vi "HW Config.vi"() -> ()   [LabVIEW 2018]
uses:
  Subvi/Global.vi
panel:
  in  "Bar":bool
  in  "退出 3":bool
  in  "另存为":bool
  in  "保存":bool
  in  "open":bool
  in  "新建":bool
  in  "delete":bool
  in  "add":bool
  out "布尔":bool
  in  "Add":bool
  in  "Tree":string(tree)="DSO-2250 USB"
  out "Ready":u8(slide) max=101 scale=0.0..100.0
  in  "File Name":string caption="文件名称"
  in  "Save As":bool
  in  "Save":bool
  in  "Multicolumn Listbox":i32(listbox)=-1
  # "添加：选中右边你要插入的行，然后双击获点击“添加(F1)”左边你的设备\n即可添加到右边所选中行的前面\n删除：选中右边你要删除的行，点击\"删除（DEL）\"\n！"
  # "DEMO:V0.0.1"
  # "ID"
  # "准备就绪"
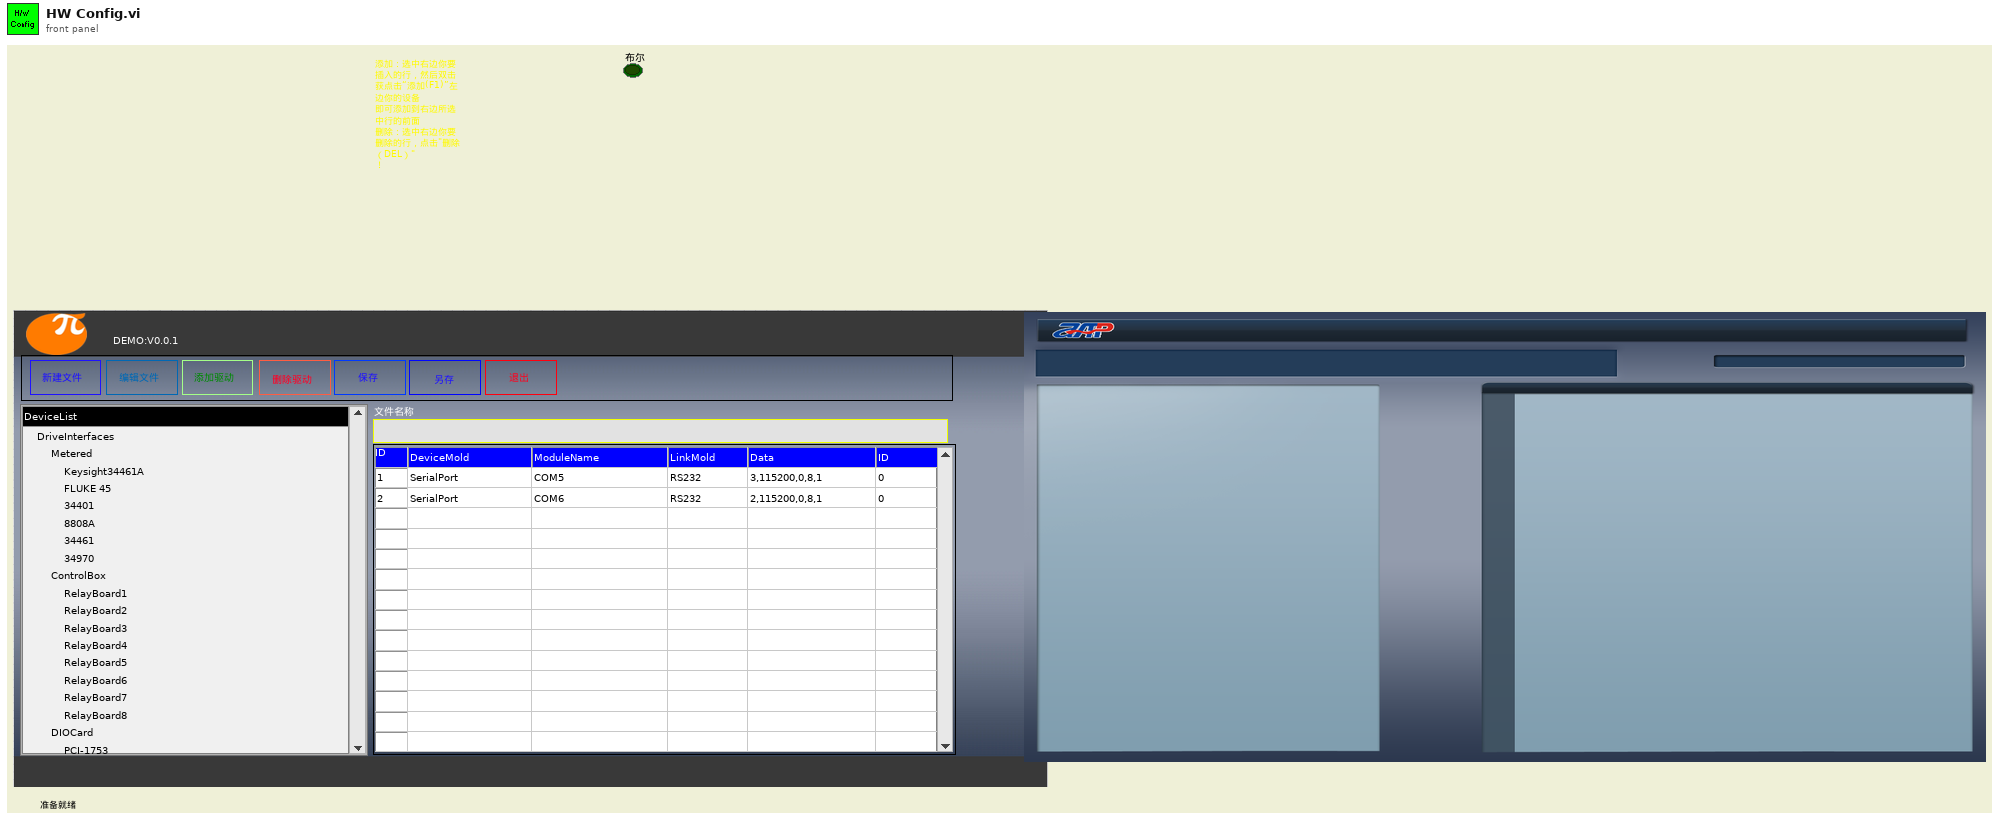
[diagram p1: front panel]
types:
  T1 = enum16{"open", "replace", "create", "open or create", "replace or create", "replace or create with confirmation"}
  T2 = typedef "Window Refnum.ctl" = refnum<k1>
  T3 = typedef "Window Rectangle.ctl" = cluster{"left":i16, "top":i16, "right":i16, "bottom":i16}
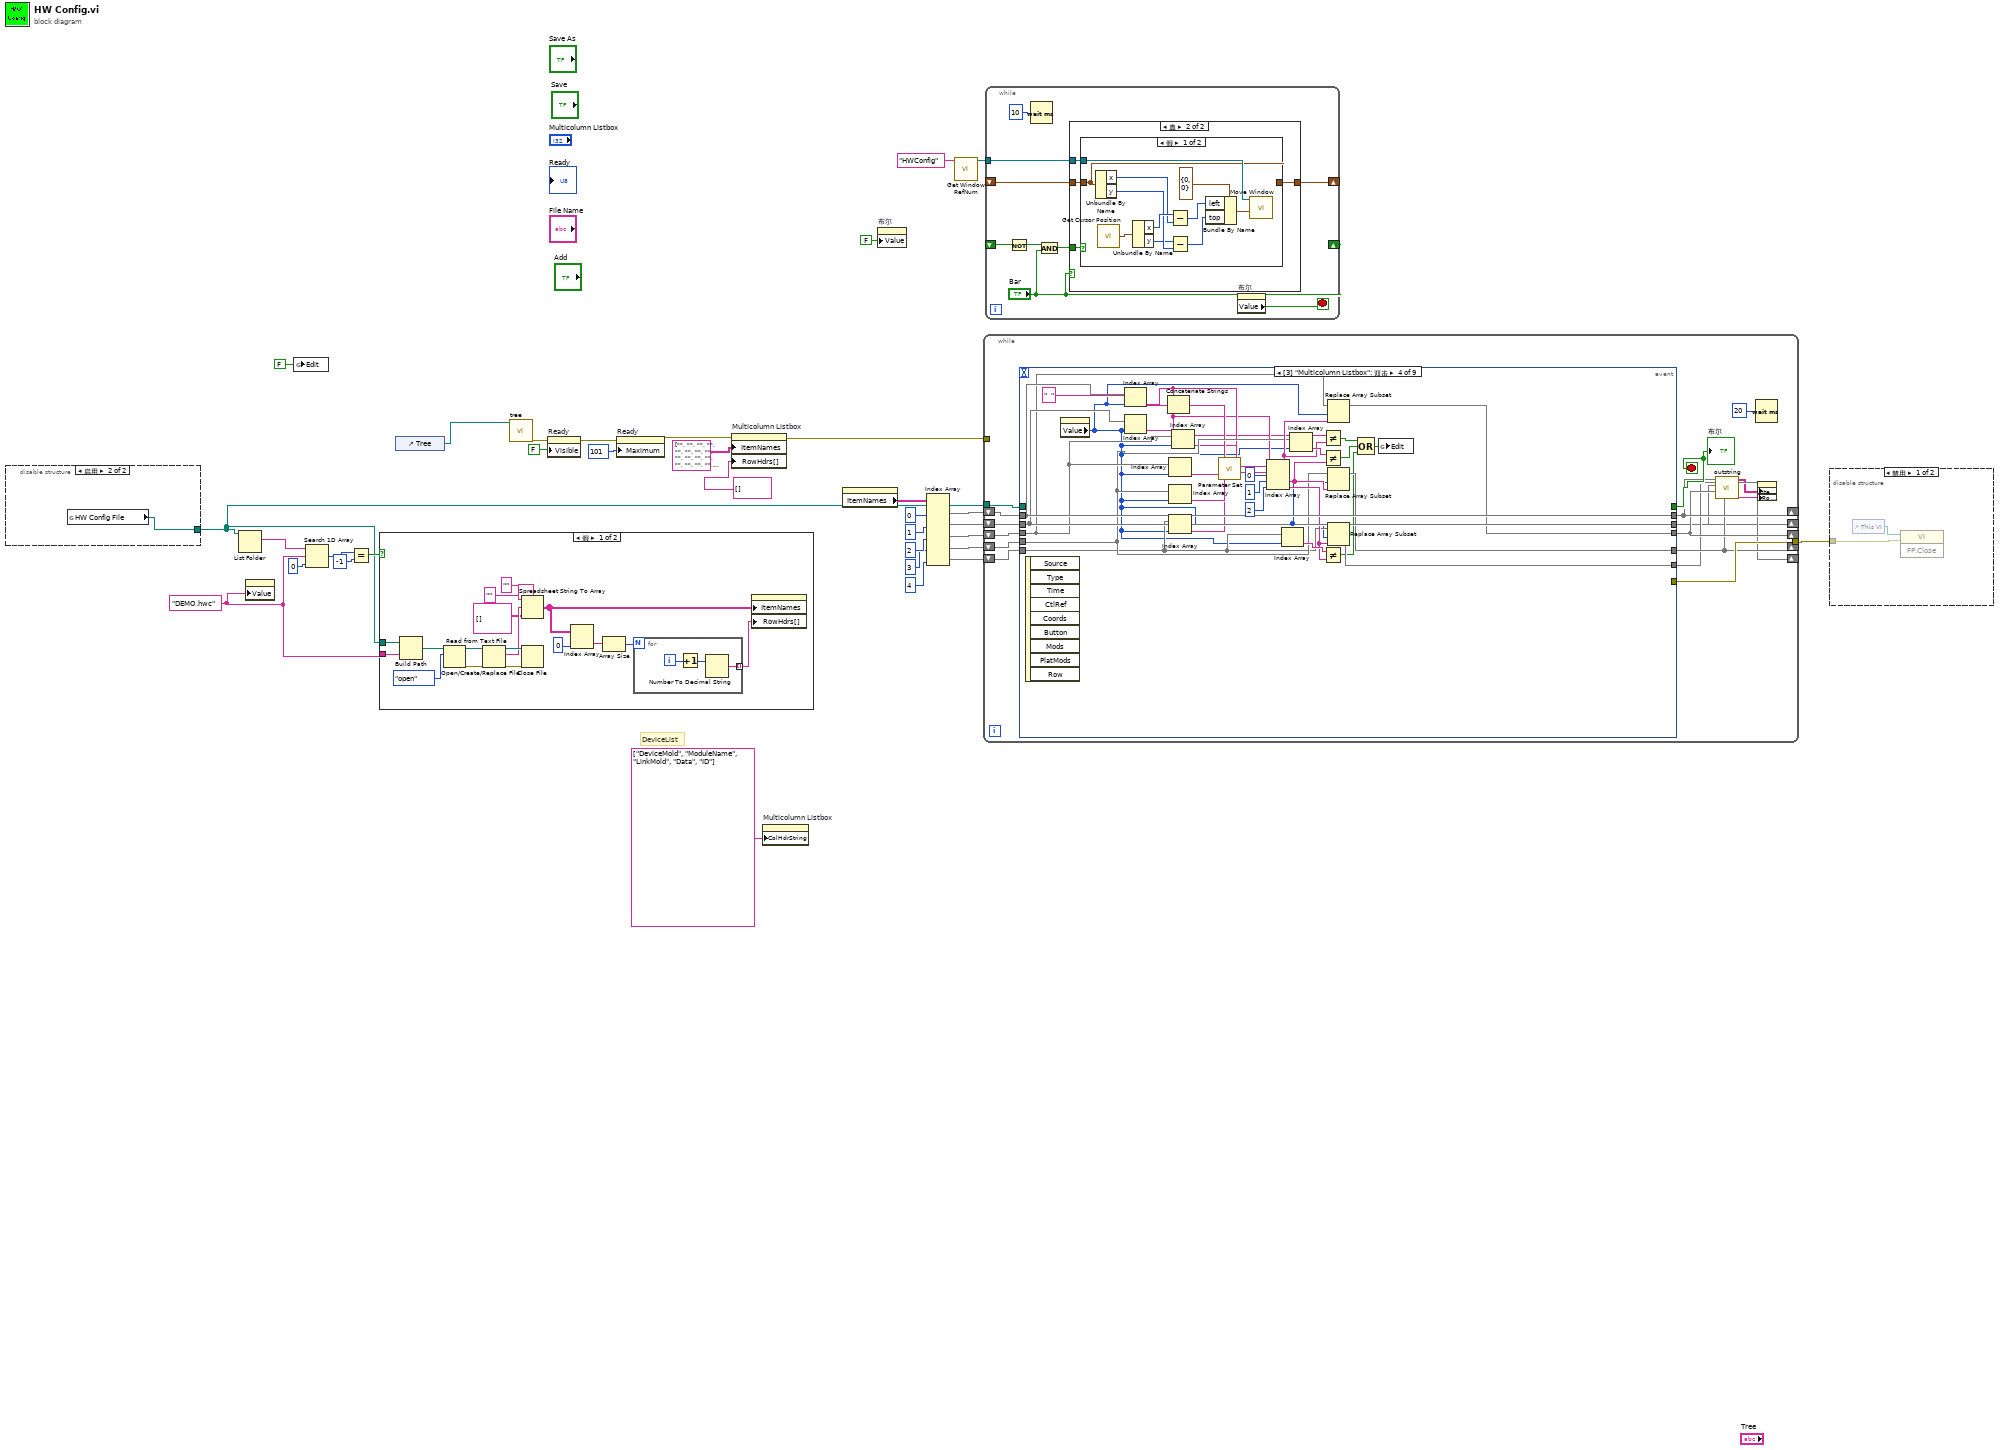
[diagram p0: block diagram]
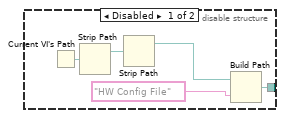
[diagram p3: hidden frame]
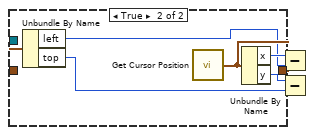
[diagram p5: hidden frame]
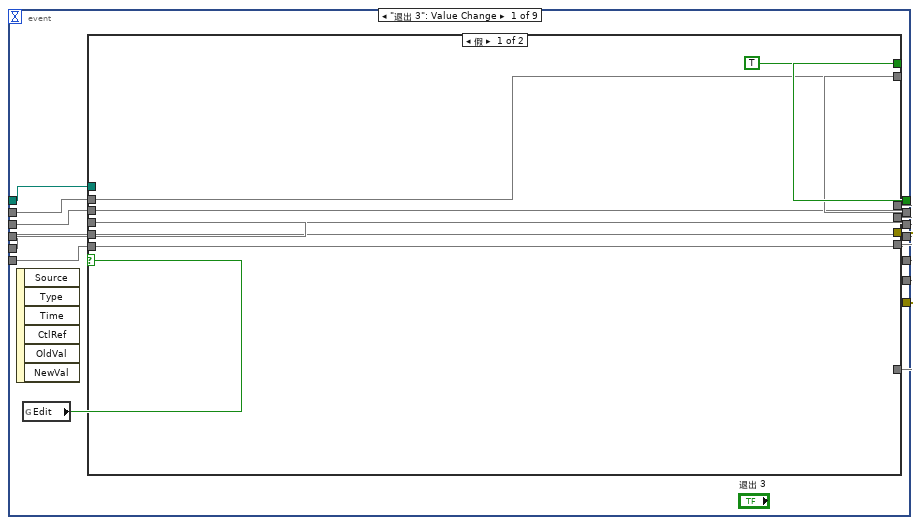
[diagram p6: hidden frame]
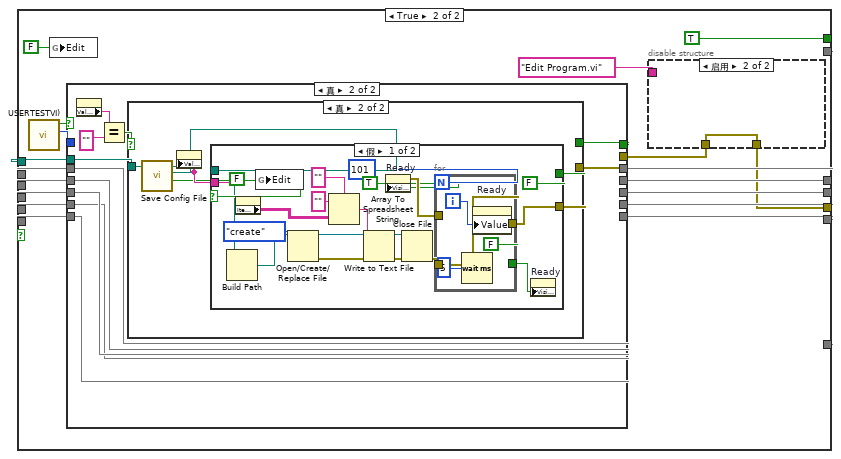
[diagram p7: hidden frame]
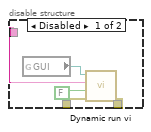
[diagram p8: hidden frame]
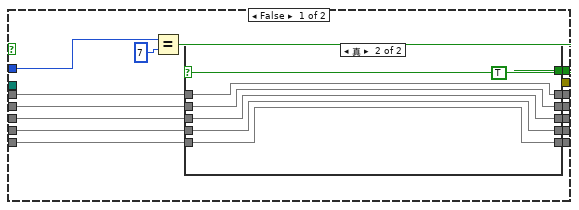
[diagram p9: hidden frame]
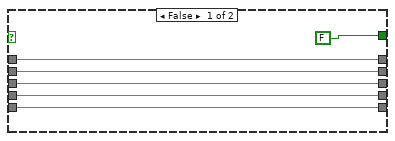
[diagram p10: hidden frame]
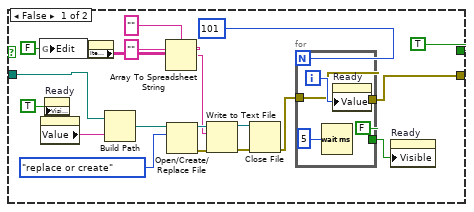
[diagram p11: hidden frame]
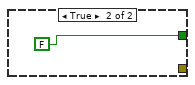
[diagram p12: hidden frame]
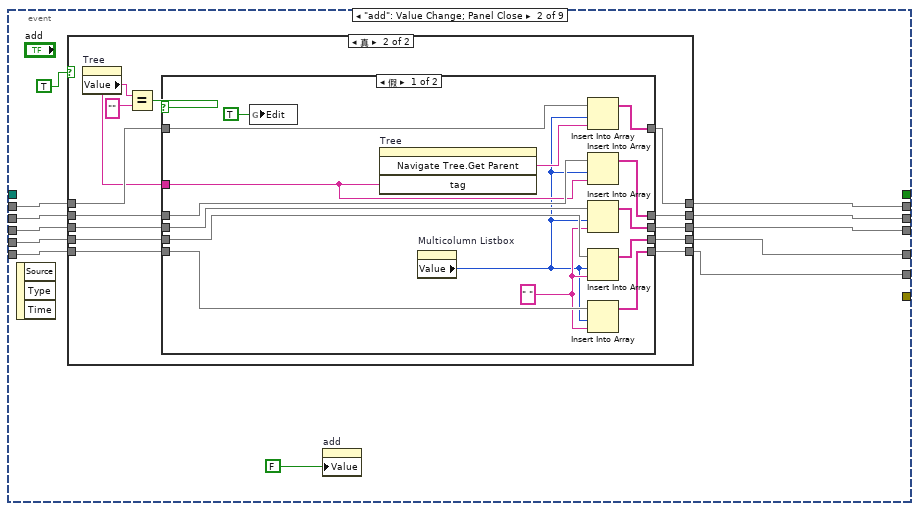
[diagram p13: hidden frame]
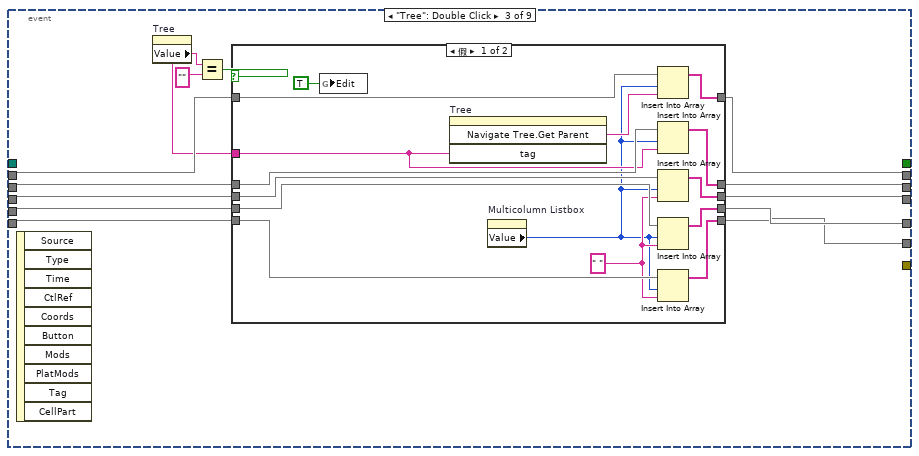
[diagram p16: hidden frame]
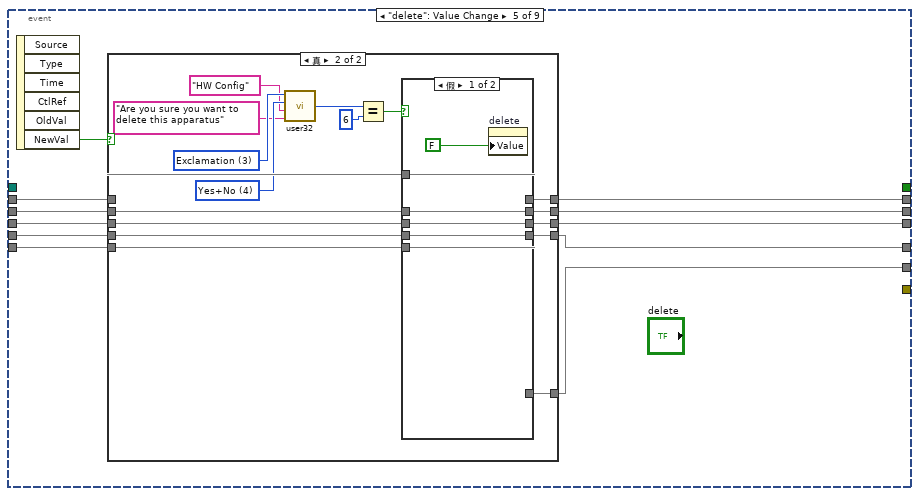
[diagram p18: hidden frame]
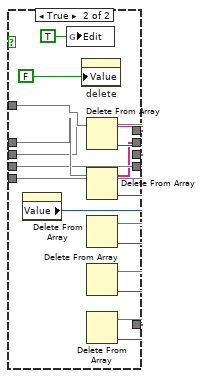
[diagram p20: hidden frame]
diagram:
  w25 = "DEMO.hwc" ("element")
  # "DeviceList"
  n1 = disable-structure shown="启用" {
    disable-tunnel: [w35 w39] -> w19
    frame Disabled {
      n2 = Current VI's Path() -> (path=w34:path)
      n3 = Strip Path(path=w34) -> (stripped path=w37:path)  [unwired: 1 out]
      n4 = Strip Path(path=w37) -> (stripped path=w38:path)  [unwired: 1 out]
      n5 = Build Path(base path=w38, name or relative path="HW Config File") -> (appended path=w35:path)
    }
    frame Enabled {
      n6 = global read "Global.vi" "HW Config File"() -> (w39:path)
    }
  }
  n7 = List Folder(path=w19) -> (filenames=w20:string[])  [unwired: 1 in, 5 out]
  n8 = property on="File Name" class="Str"("Value"=w25) -> ()  [unwired: 2 in, 2 out]
  n9 = global write "Global.vi" "Edit"(FALSE) -> ()
  n10 = Search 1D Array(1D array=w20, element=w25, start index (0)=0) -> (index of element=w22:i32)
  n11 = Equal?(x=w22, y=-1) -> (x = y?=w24:bool)
  n12 = case shown="假" w24 {
    tunnel: w19 -> [w56 w68]
    tunnel: w25 -> [w55 w67]
    frame False {
      n13 = Build Path(base path=w56, name or relative path=w55) -> (appended path=w54:path)
      n14 = Open/Create/Replace File(file path (use dialog)=w54, operation (0:open)=T1."open") -> (refnum out=w53:refnum<file>, error out=w51:errorcluster)  [unwired: 1 in, 4 out]
      n15 = Read from Text File(file (use dialog)=w53, error in=w51) -> (refnum out=w52:refnum<file>, text=w48:string, error out=w50:errorcluster)  [unwired: 3 out]
      n16 = Spreadsheet String To Array(delimiter (Tab)="", format string="", spreadsheet string=w48, array type (2D Dbl)=string[][] []) -> (array=w44:string[][])
      n17 = Close File(refnum=w52, error in=w50) -> ()  [unwired: 2 out]
      n18 = Index Array(array=w44, index (col)=0 ("disabled index (col)")) -> (element=w42:string[])  [unwired: 1 in]
      n19 = Array Size(array=w42) -> (size(s)=w41:i32)
      n20 = for {
        N: w41 -> [_]
        tunnel: [w57] -> w40 mode=indexing
        i -> [w59]
        n21 = Increment(x=w59) -> (x+1=w58:i32)
        n22 = Number To Decimal String(number=w58) -> (decimal integer string=w57:string)  [unwired: 1 out]
      }
      n23 = property on="Multicolumn Listbox" class="MCListbox (严格)"("ItemNames"=w44, "RowHdrs[]"=w40) -> ()  [unwired: 2 in, 2 out]
    }
    frame True {
      n24 = Build Path(base path=w68, name or relative path=w67) -> (appended path=w66:path)
      n25 = Open/Create/Replace File(file path (use dialog)=w66, operation (0:open)=T1."create") -> (refnum out=w64:refnum<file>, error out=w63:errorcluster)  [unwired: 1 in, 4 out]
      n26 = Write to Text File(file (use dialog)=w64, text="DC Source\tAPM\tRS 232\t2,9600,0,8,1\t1\nDC Source\tAPM\tRS 232\t3,9600,0,8,1\t2\nDC Source\tAPM\tRS 232\t4,9600,0,8,1\t3\nDC Source\tAPM\tRS 232\t5,9600,0,8,1\t4\nOscilloscope\tDSO-2250 USB\tUSB\t0\t1\nCAN Card\tGY8507\tUSB\t0\t1\nDIO Card\tPCI 1753\tPCI Card\t4\t1\nDAQ\tPCI-1713\tPCI Card\t3\t1\n", error in=w63) -> (refnum out=w62:refnum<file>, error out=w61:errorcluster)  [unwired: 2 out]
      n27 = Close File(refnum=w62, error in=w61) -> ()  [unwired: 2 out]
    }
  }
  n28 = control-ref of="Tree"() -> (w4:refnum<vi>)
  n29 = call "tree.vi"("search"=w4) -> ("error out"=w3:errorcluster)  [unwired: 9 in, 1 out]
  n30 = property on="Ready" class="Slide (严格)"(error in=w3, "Visible"=FALSE) -> (error out=w27:errorcluster)  [unwired: 1 in, 1 out]
  n31 = property on="Ready" class="Slide (严格)"(error in=w27, "Maximum"=101) -> (error out=w29:errorcluster)  [unwired: 1 in, 1 out]
  n32 = property on="Multicolumn Listbox" class="MCListbox (严格)"(error in=w29, "ItemNames"=string[][] [["", "", "", "", ""], ["", "", "", "", ""], ["", "", "", "", ""], ["", "", "", "", ""], ["", "", "", "", ""], ["", "", "", "", ""], ["", "", "", "", ""], ["", "", "", "", ""], ["", "", "", "", ""], ["", "", "", "", ""], ["", "", "", "", ""], ["", "", "", "", ""], ["", "", "", "", ""], ["", "", "", "", ""], ["", "", "", "", ""], ["", "", "", "", ""], ["", "", "", "", ""], ["", "", "", "", ""], ["", "", "", "", ""], ["", "", "", "", ""], ["", "", "", "", ""], ["", "", "", "", ""], ["", "", "", "", ""], ["", "", "", "", ""], ["", "", "", "", ""], ["", "", "", "", ""], ["", "", "", "", ""], ["", "", "", "", ""], ["", "", "", "", ""], ["", "", "", "", ""], ["", "", "", "", ""], ["", "", "", "", ""], ["", "", "", "", ""], ["", "", "", "", ""], ["", "", "", "", ""], ["", "", "", "", ""], ["", "", "", "", ""], ["", "", "", "", ""], ["", "", "", "", ""], ["", "", "", "", ""], ["", "", "", "", ""], ["", "", "", "", ""], ["", "", "", "", ""], ["", "", "", "", ""], ["", "", "", "", ""]], "RowHdrs[]"=string[] []) -> (error out=w7:errorcluster)  [unwired: 1 in, 1 out]
  n33 = property on="Multicolumn Listbox" class="MCListbox (严格)"("ColHdrString"=string[] ["DeviceMold", "ModuleName", "LinkMold", "Data", "ID"] ("Column Header Strings[]")) -> ()  [unwired: 2 in, 2 out]
  n34 = property on="Multicolumn Listbox" class="MCListbox (严格)"() -> ("ItemNames"=w18:string[][])  [unwired: 2 in, 2 out]
  n35 = property on="布尔" class="Bool (严格)"("Value"=FALSE ("布尔")) -> ()  [unwired: 2 in, 2 out]
  n36 = Index Array(array=w18, index (col) #1=0 ("disabled index (col)"), index (col) #2=1 ("index (col)"), index (col) #3=2 ("index (col)"), index (col) #4=3 ("index (col)"), index (col) #5=4 ("index (col)")) -> (element #1=w12:string[], element #2=w11:string[], element #3=w10:string[], element #4=w9:string[], element #5=w8:string[])  [unwired: 5 in]
  n37 = call "Get Window RefNum.vi"("window name (\"\")"="HWConfig" ("window name (\"\")")) -> ("window refnum (NaWR)"=w6:T2)  [unwired: 1 in, 7 out]
  n38 = while {
    tunnel: [w83] -> w32
    shift-right: [w79] -> _
    shift-left: w12 -> [w74]
    shift-right: [w71] -> _
    shift-left: w11 -> [w73]
    shift-right: [w78] -> _
    shift-left: w10 -> [w81]
    shift-right: [w77] -> _
    shift-left: w9 -> [w72]
    shift-right: [w76] -> _
    shift-left: w8 -> [w80]
    tunnel: w19 -> [w69]
    tunnel: w7 -> [_]
    stop <- w82 stop-if-true
    n39 = event shown="[3] \"Multicolumn Listbox\": 双击" {
      selector: _ -> [_ _ _ _ _ _ _ _ _]
      dyn-events: _ -> [_ _ _ _ _ _ _ _ _]
      timeout: _ -> [_ _ _ _ _ _ _ _ _]
      tunnel: [w96 _ _ _ _ _ _ w473 _] -> w83
      tunnel: [w95 _ _ _ _ _ _ _ _] -> w82
      tunnel: w81 -> [w92 w223 w279 w313 w340 w390 w443 _ w504]
      tunnel: w80 -> [w90 w227 w277 w311 w338 w388 w441 _ w502]
      tunnel: [w89 w229 w276 w327 w337 w392 w445 w478 w513] -> w79
      tunnel: [w88 w228 w275 w326 w336 w391 w444 w477 w512] -> w71
      tunnel: [w87 w222 w274 w325 w335 w390 w443 w476 w511] -> w78
      tunnel: [w86 w220 w273 w324 w334 w389 w442 w475 w510] -> w77
      tunnel: [w85 w226 w272 w323 w333 w388 w441 w474 w509] -> w76
      tunnel: w74 -> [w94 w230 w281 w327 w342 w392 w445 _ w506]
      tunnel: w73 -> [w93 w224 w280 w326 w341 w391 w444 _ w505]
      tunnel: w72 -> [w91 w221 w278 w312 w339 w389 w442 _ w503]
      tunnel: w69 -> [w97 _ _ _ _ w387 w447 w489 w514]
      event "退出 3": Value Change {
        n40 = event-data() -> ()  [unwired: 7 out]
        n41 = global read "Global.vi" "Edit"() -> (w98:bool)
        n42 = case shown="假" w98 {
          tunnel: w97 -> [_ w121]
          tunnel: [_ w106] -> w96
          tunnel: [TRUE TRUE] -> w95
          tunnel: [w103 w114] -> w89
          tunnel: w94 -> [w103 w119]
          tunnel: [w102 w113] -> w88
          tunnel: w93 -> [w102 w118]
          tunnel: [w101 w112] -> w87
          tunnel: w92 -> [w101 w117]
          tunnel: [w100 w111] -> w86
          tunnel: w91 -> [w100 w116]
          tunnel: [w99 w110] -> w85
          tunnel: w90 -> [w99 w115]
          frame False {
          }
          frame True {
            n43 = call "USERTESTVI).vi"() -> ("buttin pressed"=w120:i32, "布尔"=w122:bool)  [unwired: 10 in]
            n44 = global write "Global.vi" "Edit"(FALSE) -> ()
            n45 = case shown="真" w122 {
              tunnel: w121 -> [_ w160]
              tunnel: w120 -> [w142 _]
              tunnel: [_ w155] -> w105
              tunnel: [w139 w156] -> _
              tunnel: [w134 w165] -> w114
              tunnel: w119 -> [w129 w165]
              tunnel: [w133 w164] -> w113
              tunnel: w118 -> [w138 w164]
              tunnel: [w132 w163] -> w112
              tunnel: w117 -> [w137 w163]
              tunnel: [w131 w162] -> w111
              tunnel: w116 -> [w136 w162]
              tunnel: [w130 w161] -> w110
              tunnel: w115 -> [w135 w161]
              frame False {
                n46 = Equal?(x=w142, y=7) -> (x = y?=w140:bool)
                n47 = case shown="真" w140 {
                  tunnel: [FALSE TRUE] -> w139
                  tunnel: [w147 w153] -> w134
                  tunnel: w129 -> [w147 w153]
                  tunnel: [w146 w152] -> w133
                  tunnel: w138 -> [w146 w152]
                  tunnel: [w145 w151] -> w132
                  tunnel: w137 -> [w145 w151]
                  tunnel: [w144 w150] -> w131
                  tunnel: w136 -> [w144 w150]
                  tunnel: [w143 w149] -> w130
                  tunnel: w135 -> [w143 w149]
                  frame False {
                  }
                  frame True {
                  }
                }
              }
              frame True {
                n48 = property on="File Name" class="Str"() -> ("Value"=w158:string)  [unwired: 2 in, 2 out]
                n49 = Equal?(x=w158, y="") -> (x = y?=w159:bool)
                n50 = case shown="真" w159 {
                  tunnel: w160 -> [w183 w193]
                  tunnel: [TRUE w191] -> w156
                  tunnel: [w166 w189] -> w155
                  frame False {
                    n51 = global write "Global.vi" "Edit"(FALSE) -> ()
                    n52 = property on="File Name" class="Str"() -> ("Value"=w182:string)  [unwired: 2 in, 2 out]
                    n53 = property on="Ready" class="Slide (严格)"("Visible"=TRUE) -> ()  [unwired: 2 in, 2 out]
                    n54 = property on="Multicolumn Listbox" class="MCListbox (严格)"() -> ("ItemNames"=w176:string[][])  [unwired: 2 in, 2 out]
                    n55 = Build Path(base path=w183, name or relative path=w182) -> (appended path=w184:path)
                    n56 = Array To Spreadsheet String(delimiter (Tab)="", array=w176, 3:"" ("format string")) -> (spreadsheet string=w173:string)
                    n57 = Open/Create/Replace File(file path (use dialog)=w184, operation (0:open)=T1."replace or create") -> (refnum out=w180:refnum<file>, error out=w181:errorcluster)  [unwired: 1 in, 4 out]
                    n58 = Write to Text File(file (use dialog)=w180, text=w173, error in=w181) -> (refnum out=w179:refnum<file>, error out=w178:errorcluster)  [unwired: 2 out]
                    n59 = Close File(refnum=w179, error in=w178) -> (error out=w167:errorcluster)  [unwired: 1 out]
                    n60 = for {
                      N: 101 -> [_]
                      tunnel: [FALSE] -> w170
                      tunnel: [w185] -> w166
                      tunnel: w167 -> [w185]
                      i -> [w188]
                      n61 = Wait (ms)(milliseconds to wait=u32 5) -> ()  [unwired: 1 out]
                      n62 = property on="Ready" class="Slide (严格)"("Value"=w188) -> ()  [unwired: 2 in, 2 out]
                    }
                    n63 = property on="Ready" class="Slide (严格)"("Visible"=w170) -> ()  [unwired: 2 in, 2 out]
                  }
                  frame True {
                    n64 = call "Save Config File.vi"("base path"=w193) -> ("Cancel"=w190:bool, "new file name"=w192:string)  [unwired: 9 out]
                    n65 = property on="File Name" class="Str"("Value"=w192) -> ()  [unwired: 2 in, 2 out]
                    n66 = case shown="假" w190 {
                      tunnel: w193 -> [w204 _]
                      tunnel: w192 -> [w203 _]
                      tunnel: [FALSE FALSE] -> w191
                      tunnel: [w194 _] -> w189
                      frame False {
                        n67 = Build Path(base path=w204, name or relative path=w203) -> (appended path=w212:path)
                        n68 = property on="Multicolumn Listbox" class="MCListbox (严格)"() -> ("ItemNames"=w213:string[][])  [unwired: 2 in, 2 out]
                        n69 = global write "Global.vi" "Edit"(FALSE) -> ()
                        n70 = Open/Create/Replace File(file path (use dialog)=w212, operation (0:open)=T1."create") -> (refnum out=w211:refnum<file>, error out=w210:errorcluster)  [unwired: 1 in, 4 out]
                        n71 = Array To Spreadsheet String(delimiter (Tab)="", array=w213, 3:"") -> (spreadsheet string=w209:string)
                        n72 = Write to Text File(file (use dialog)=w211, text=w209, error in=w210) -> (refnum out=w208:refnum<file>, error out=w207:errorcluster)  [unwired: 2 out]
                        n73 = property on="Ready" class="Slide (严格)"("Visible"=TRUE) -> (error out=w199:errorcluster)  [unwired: 2 in, 1 out]
                        n74 = Close File(refnum=w208, error in=w207) -> (error out=w195:errorcluster)  [unwired: 1 out]
                        n75 = for {
                          N: 101 -> [_]
                          tunnel: w199 -> [_]
                          tunnel: [FALSE] -> w197
                          tunnel: w195 -> [w214]
                          tunnel: [w214] -> w194
                          i -> [w217]
                          n76 = Wait (ms)(milliseconds to wait=u32 5) -> ()  [unwired: 1 out]
                          n77 = property on="Ready" class="Slide (严格)"("Value"=w217) -> ()  [unwired: 2 in, 2 out]
                        }
                        n78 = property on="Ready" class="Slide (严格)"("Visible"=w197) -> ()  [unwired: 2 in, 2 out]
                      }
                      frame True {
                      }
                    }
                  }
                }
              }
            }
            n79 = disable-structure shown="启用" {
              disable-tunnel: "Edit Program.vi" ("vi name") -> [w127 _]
              disable-tunnel: [w125 w128] -> w106
              disable-tunnel: w105 -> [w124 w128]
              frame Disabled {
                n80 = global read "Global.vi" "GUI"() -> (w123:path)
                n81 = call "Dynamic run vi.vi"("error in (no error)"=w124, "Wait Until Done"=FALSE, "vi name"=w127, "path"=w123) -> ("error out"=w125:errorcluster)  [unwired: 4 out]
              }
              frame Enabled {
              }
            }
          }
        }
      }
      event "add": Value Change; Panel Close {
        n82 = event-data() -> ()  [unwired: 4 out]
        n83 = case shown="真" TRUE {
          tunnel: w230 -> [w235 w248]
          tunnel: [w235 w247] -> w229
          tunnel: [w234 w246] -> w228
          tunnel: w227 -> [w231 w245]
          tunnel: [w231 w244] -> w226
          tunnel: w224 -> [w234 w243]
          tunnel: w223 -> [w233 w242]
          tunnel: [w233 w241] -> w222
          tunnel: w221 -> [w232 w240]
          tunnel: [w232 w239] -> w220
          frame False {
          }
          frame True {
            n84 = property on="Tree" class="Tree (严格)"() -> ("Value"=w236:string)  [unwired: 2 in, 2 out]
            n85 = Equal?(x=w236, y="") -> (x = y?=w237:bool)
            n86 = case shown="假" w237 {
              tunnel: w248 -> [w263 w268]
              tunnel: [w262 w268] -> w247
              tunnel: [w261 w267] -> w246
              tunnel: w245 -> [w254 w264]
              tunnel: [w252 w264] -> w244
              tunnel: w243 -> [w256 w267]
              tunnel: w242 -> [w260 w266]
              tunnel: [w259 w266] -> w241
              tunnel: w240 -> [w258 w265]
              tunnel: [w257 w265] -> w239
              tunnel: w236 -> [w251 _]
              frame False {
                w253 = " "
                n87 = global write "Global.vi" "Edit"(TRUE) -> ()
                n88 = invoke on="Tree" class="Tree (strict)" method="Navigate Tree.Get Parent"("tag"=w251) -> ("Navigate Tree:Get Parent"=w250:string)  [unwired: 3 in, 3 out]
                n89 = property on="Multicolumn Listbox" class="MCListbox (严格)"() -> ("Value"=w249:i32)  [unwired: 2 in, 2 out]
                n90 = Insert Into Array(array=w263, index=w249, new element=w250) -> (w262:string[])
                n91 = Insert Into Array(array=w256, index=w249, new element=w251) -> (w261:string[])
                n92 = Insert Into Array(array=w260, index=w249, new element=w253) -> (w259:string[])
                n93 = Insert Into Array(array=w258, index=w249, new element=w253) -> (w257:string[])
                n94 = Insert Into Array(array=w254, index=w249, new element=w253) -> (w252:string[])
              }
              frame True {
              }
            }
          }
        }
        n95 = property on="add" class="Bool (严格)"("Value"=FALSE) -> ()  [unwired: 2 in, 2 out]
      }
      event "Tree": Double Click {
        n96 = event-data() -> ()  [unwired: 11 out]
        n97 = property on="Tree" class="Tree (严格)"() -> ("Value"=w269:string)  [unwired: 2 in, 2 out]
        n98 = Equal?(x=w269, y="") -> (x = y?=w270:bool)
        n99 = case shown="假" w270 {
          tunnel: w281 -> [w296 w301]
          tunnel: [w295 w301] -> w276
          tunnel: [w294 w300] -> w275
          tunnel: w277 -> [w287 w297]
          tunnel: [w285 w297] -> w272
          tunnel: w280 -> [w289 w300]
          tunnel: w279 -> [w293 w299]
          tunnel: [w292 w299] -> w274
          tunnel: w278 -> [w291 w298]
          tunnel: [w290 w298] -> w273
          tunnel: w269 -> [w284 _]
          frame False {
            w286 = " "
            n100 = global write "Global.vi" "Edit"(TRUE) -> ()
            n101 = invoke on="Tree" class="Tree (strict)" method="Navigate Tree.Get Parent"("tag"=w284) -> ("Navigate Tree:Get Parent"=w283:string)  [unwired: 3 in, 3 out]
            n102 = property on="Multicolumn Listbox" class="MCListbox (严格)"() -> ("Value"=w282:i32)  [unwired: 2 in, 2 out]
            n103 = Insert Into Array(array=w296, index=w282, new element=w283) -> (w295:string[])
            n104 = Insert Into Array(array=w289, index=w282, new element=w284) -> (w294:string[])
            n105 = Insert Into Array(array=w293, index=w282, new element=w286) -> (w292:string[])
            n106 = Insert Into Array(array=w291, index=w282, new element=w286) -> (w290:string[])
            n107 = Insert Into Array(array=w287, index=w282, new element=w286) -> (w285:string[])
          }
          frame True {
          }
        }
      }
      event "Multicolumn Listbox": Double Click {
        n108 = event-data() -> ()  [unwired: 10 out]
        n109 = property on="Multicolumn Listbox" class="MCListbox (严格)"() -> ("Value"=w302:i32)  [unwired: 2 in, 2 out]
        n110 = Index Array(array=w327, index=w302) -> (element=w305:string)
        n111 = Index Array(array=w326, index=w302) -> (element=w304:string)
        n112 = Concatenate Strings(w305, "  " ("string"), w304) -> (w310:string)
        n113 = Index Array(array=w313, index=w302) -> (element=w308:string)
        n114 = Index Array(array=w312, index=w302) -> (element=w307:string)
        n115 = Index Array(array=w311, index=w302) -> (element=w306:string)
        n116 = Index Array(array=w313, index=w302) -> (element=w303:string)
        n117 = call "Parameter Set.vi"("Device Type"=w305, "Model Name"=w304, 3:"Interface"=w303, "Index Num"=w306, "Parameter"=w307, 6:"Interface"=w308, "Model"=w310) -> ("Data out"=w309:string[])
        n118 = Index Array(array=w309, index #1=0, index #2=1, index #3=2) -> (element #1=w320:string, element #2=w319:string, element #3=w318:string)
        n119 = Index Array(array=w311, index=w302) -> (element=w321:string)
        n120 = Index Array(array=w312, index=w302) -> (element=w322:string)
        n121 = Not Equal?(x=w303, y=w320) -> (x != y?=w317:bool)
        n122 = Not Equal?(x=w322, y=w319) -> (x != y?=w316:bool)
        n123 = Not Equal?(x=w321, y=w318) -> (x != y?=w315:bool)
        n124 = Replace Array Subset(array=w313, new element=w320, index=w302) -> (w325:string[])
        n125 = Replace Array Subset(array=w312, new element=w319, index=w302) -> (w324:string[])
        n126 = Replace Array Subset(array=w311, new element=w318, index=w302) -> (w323:string[])
        n127 = Compound Arithmetic op=OR(w317, w316, w315) -> (w314:bool)
        n128 = global write "Global.vi" "Edit"(w314) -> ()
      }
      event "delete": Value Change {
        n129 = event-data() -> ("NewVal"=w332:bool)  [unwired: 6 out]
        n130 = case shown="真" w332 {
          tunnel: w342 -> [w343 w364]
          tunnel: w341 -> [w347 w363]
          tunnel: w340 -> [w346 w362]
          tunnel: w339 -> [w345 w361]
          tunnel: w338 -> [w344 w360]
          tunnel: [w343 w359] -> w337
          tunnel: [w347 w358] -> w336
          tunnel: [w346 w357] -> w335
          tunnel: [w345 w356] -> w334
          tunnel: [w344 w355] -> w333
          frame False {
          }
          frame True {
            w353 = u16 4 items=["OK", "OK+Cancel", "Abort+Retry+Ignore", "Yes+ON+Cancel", "Yes+No", "Retry+Cancel", "Cancel+Retry+Continue"] ("Buttons")
            w354 = u16 3 items=["None", "Critical", "Question", "Exclamation", "Infomation"] ("Icon")
            n131 = call "user32.vi"("Icon"=w354, "Buttons"=w353, "Ipcaption"="HW Config", "IP Text"="Are you sure you want to delete this apparatus") -> ("buttin pressed"=w350:i32)  [unwired: 1 out]
            n132 = Equal?(x=w350, y=6) -> (x = y?=w348:bool)
            n133 = case shown="假" w348 {
              tunnel: w364 -> [w370 w383]
              tunnel: w363 -> [w366 w382]
              tunnel: w362 -> [w369 w381]
              tunnel: w361 -> [w368 w380]
              tunnel: w360 -> [w367 w379]
              tunnel: [w370 w377] -> w359
              tunnel: [w366 w373] -> w358
              tunnel: [w369 w376] -> w357
              tunnel: [w368 w375] -> w356
              tunnel: [w367 w374] -> w355
              frame False {
                n134 = property on="delete" class="Bool (严格)"("Value"=FALSE) -> ()  [unwired: 2 in, 2 out]
              }
              frame True {
                n135 = property on="Multicolumn Listbox" class="MCListbox (严格)"() -> ("Value"=w378:i32)  [unwired: 2 in, 2 out]
                n136 = global write "Global.vi" "Edit"(TRUE) -> ()
                n137 = property on="delete" class="Bool (严格)"("Value"=FALSE) -> ()  [unwired: 2 in, 2 out]
                n138 = Delete From Array(array=w383, index=w378) -> (array with subset deleted=w377:string[])  [unwired: 1 in, 1 out]
                n139 = Delete From Array(array=w382, index=w378) -> (array with subset deleted=w373:string[])  [unwired: 1 in, 1 out]
                n140 = Delete From Array(array=w381, index=w378) -> (array with subset deleted=w376:string[])  [unwired: 1 in, 1 out]
                n141 = Delete From Array(array=w380, index=w378) -> (array with subset deleted=w375:string[])  [unwired: 1 in, 1 out]
                n142 = Delete From Array(array=w379, index=w378) -> (array with subset deleted=w374:string[])  [unwired: 1 in, 1 out]
              }
            }
          }
        }
      }
      event "保存": Value Change {
        n143 = event-data() -> ()  [unwired: 7 out]
        n144 = property on="File Name" class="Str"() -> ("Value"=w384:string)  [unwired: 2 in, 2 out]
        n145 = Equal?(x=w384, y="") -> (x = y?=w385:bool)
        n146 = case shown="真" w385 {
          tunnel: w387 -> [w394 w415]
          tunnel: w384 -> [w393 _]
          frame False {
            n147 = global write "Global.vi" "Edit"(FALSE) -> ()
            n148 = Build Path(base path=w394, name or relative path=w393) -> (appended path=w411:path)
            n149 = property on="Ready" class="Slide (严格)"("Visible"=TRUE) -> (error out=w397:errorcluster)  [unwired: 2 in, 1 out]
            n150 = property on="Multicolumn Listbox" class="MCListbox (严格)"() -> ("ItemNames"=w406:string[][])  [unwired: 2 in, 2 out]
            n151 = for {
              N: 101 -> [_]
              tunnel: w397 -> [_]
              tunnel: [FALSE] -> w395
              i -> [w414]
              n152 = Wait (ms)(milliseconds to wait=u32 5) -> ()  [unwired: 1 out]
              n153 = property on="Ready" class="Slide (严格)"("Value"=w414) -> ()  [unwired: 2 in, 2 out]
            }
            n154 = Array To Spreadsheet String(delimiter (Tab)="", array=w406, 3:"" ("format string")) -> (spreadsheet string=w403:string)
            n155 = Open/Create/Replace File(file path (use dialog)=w411, operation (0:open)=T1."replace or create") -> (refnum out=w410:refnum<file>, error out=w409:errorcluster)  [unwired: 1 in, 4 out]
            n156 = Write to Text File(file (use dialog)=w410, text=w403, error in=w409) -> (refnum out=w408:refnum<file>, error out=w407:errorcluster)  [unwired: 2 out]
            n157 = Close File(refnum=w408, error in=w407) -> (error out=w401:errorcluster)  [unwired: 1 out]
            n158 = property on="Ready" class="Slide (严格)"("Visible"=w395) -> ()  [unwired: 2 in, 2 out]
            n159 = property on="保存" class="Bool (严格)"(error in=w401, "Value"=FALSE) -> ()  [unwired: 1 in, 2 out]
          }
          frame True {
            n160 = call "Save Config File.vi"("base path"=w415) -> ("Cancel"=w417:bool, "new file name"=w416:string)  [unwired: 9 out]
            n161 = case shown="假" w417 {
              tunnel: w416 -> [w418 _]
              tunnel: w415 -> [w435 _]
              frame False {
                n162 = property on="File Name" class="Str"("Value"=w418) -> ()  [unwired: 2 in, 2 out]
                n163 = global write "Global.vi" "Edit"(FALSE) -> ()
                n164 = Build Path(base path=w435, name or relative path=w418) -> (appended path=w436:path)
                n165 = property on="Multicolumn Listbox" class="MCListbox (严格)"() -> ("ItemNames"=w430:string[][])  [unwired: 2 in, 2 out]
                n166 = Array To Spreadsheet String(delimiter (Tab)="", array=w430, 3:"" ("format string")) -> (spreadsheet string=w427:string)
                n167 = property on="Ready" class="Slide (严格)"("Visible"=TRUE) -> (error out=w421:errorcluster)  [unwired: 2 in, 1 out]
                n168 = Open/Create/Replace File(file path (use dialog)=w436, operation (0:open)=T1."open or create") -> (refnum out=w434:refnum<file>, error out=w433:errorcluster)  [unwired: 1 in, 4 out]
                n169 = for {
                  N: 101 -> [_]
                  tunnel: w421 -> [_]
                  tunnel: [FALSE] -> w419
                  i -> [w439]
                  n170 = Wait (ms)(milliseconds to wait=u32 5) -> ()  [unwired: 1 out]
                  n171 = property on="Ready" class="Slide (严格)"("Value"=w439) -> ()  [unwired: 2 in, 2 out]
                }
                n172 = Write to Text File(file (use dialog)=w434, text=w427, error in=w433) -> (refnum out=w432:refnum<file>, error out=w431:errorcluster)  [unwired: 2 out]
                n173 = Close File(refnum=w432, error in=w431) -> (error out=w425:errorcluster)  [unwired: 1 out]
                n174 = property on="保存" class="Bool (严格)"(error in=w425, "Value"=FALSE) -> ()  [unwired: 1 in, 2 out]
                n175 = property on="Ready" class="Slide (严格)"("Visible"=w419) -> ()  [unwired: 2 in, 2 out]
              }
              frame True {
                n176 = property on="保存" class="Bool (严格)"("Value"=FALSE) -> ()  [unwired: 2 in, 2 out]
              }
            }
          }
        }
      }
      event "另存为": Value Change {
        n177 = call "Save Config File.vi"("base path"=w447) -> ("Cancel"=w448:bool, "new file name"=w446:string)  [unwired: 9 out]
        n178 = event-data() -> ()  [unwired: 7 out]
        n179 = case shown="假" w448 {
          tunnel: w446 -> [w451 _]
          tunnel: w447 -> [w465 _]
          frame False {
            n180 = property on="File Name" class="Str"("Value"=w451) -> ()  [unwired: 2 in, 2 out]
            n181 = property on="Multicolumn Listbox" class="MCListbox (严格)"() -> ("ItemNames"=w460:string[][])  [unwired: 2 in, 2 out]
            n182 = property on="Ready" class="Slide (严格)"("Visible"=TRUE) -> (error out=w454:errorcluster)  [unwired: 2 in, 1 out]
            n183 = Build Path(base path=w465, name or relative path=w451) -> (appended path=w466:path)
            n184 = Array To Spreadsheet String(delimiter (Tab)="", array=w460, 3:"" ("format string")) -> (spreadsheet string=w457:string)
            n185 = Open/Create/Replace File(file path (use dialog)=w466, operation (0:open)=T1."open or create") -> (refnum out=w464:refnum<file>, error out=w463:errorcluster)  [unwired: 1 in, 4 out]
            n186 = for {
              N: 101 -> [_]
              tunnel: w454 -> [_]
              tunnel: [FALSE] -> w452
              i -> [w469]
              n187 = Wait (ms)(milliseconds to wait=u32 5) -> ()  [unwired: 1 out]
              n188 = property on="Ready" class="Slide (严格)"("Value"=w469) -> ()  [unwired: 2 in, 2 out]
            }
            n189 = Write to Text File(file (use dialog)=w464, text=w457, error in=w463) -> (refnum out=w462:refnum<file>, error out=w461:errorcluster)  [unwired: 2 out]
            n190 = Close File(refnum=w462, error in=w461) -> (error out=w450:errorcluster)  [unwired: 1 out]
            n191 = property on="Ready" class="Slide (严格)"("Visible"=w452) -> ()  [unwired: 2 in, 2 out]
            n192 = property on="另存为" class="Bool (严格)"(error in=w450, "Value"=FALSE) -> ()  [unwired: 1 in, 2 out]
          }
          frame True {
            n193 = property on="另存为" class="Bool (严格)"("Value"=FALSE) -> ()  [unwired: 2 in, 2 out]
          }
        }
      }
      event "新建": Value Change {
        n194 = event-data() -> ()  [unwired: 7 out]
        n195 = call "Save Config File.vi"("base path"=w489) -> ("new file name"=w488:string)  [unwired: 10 out]
        n196 = property on="Multicolumn Listbox" class="MCListbox (严格)"("ItemNames"=string[][] [["NA", "N", "N", "N", "N"], ["", "", "", "", ""], ["", "", "", "", ""], ["", "", "", "", ""], ["", "", "", "", ""], ["", "", "", "", ""], ["", "", "", "", ""], ["", "", "", "", ""], ["", "", "", "", ""], ["", "", "", "", ""], ["", "", "", "", ""], ["", "", "", "", ""], ["", "", "", "", ""], ["", "", "", "", ""], ["", "", "", "", ""], ["", "", "", "", ""], ["", "", "", "", ""], ["", "", "", "", ""], ["", "", "", "", ""], ["", "", "", "", ""], ["", "", "", "", ""], ["", "", "", "", ""], ["", "", "", "", ""], ["", "", "", "", ""], ["", "", "", "", ""], ["", "", "", "", ""], ["", "", "", "", ""], ["", "", "", "", ""], ["", "", "", "", ""], ["", "", "", "", ""], ["", "", "", "", ""], ["", "", "", "", ""], ["", "", "", "", ""], ["", "", "", "", ""], ["", "", "", "", ""], ["", "", "", "", ""], ["", "", "", "", ""], ["", "", "", "", ""], ["", "", "", "", ""], ["", "", "", "", ""], ["", "", "", "", ""], ["", "", "", "", ""], ["", "", "", "", ""], ["", "", "", "", ""], ["", "", "", "", ""]], "RowHdrs[]"=string[] ["1"]) -> (error out=w472:errorcluster)  [unwired: 2 in, 1 out]
        n197 = property on="File Name" class="Str"(error in=w472, "Value"=w488) -> ()  [unwired: 1 in, 2 out]
        n198 = disable-structure shown="禁用" {
          disable-tunnel: w489 -> [w500 _]
          disable-tunnel: w488 -> [w499 _]
          disable-tunnel: [w494 _] -> w473
          frame Disabled {
            n199 = Build Path(base path=w500, name or relative path=w499) -> (appended path=w498:path)
            n200 = Open/Create/Replace File(file path (use dialog)=w498) -> (refnum out=w493:refnum<file>, error out=w492:errorcluster)  [unwired: 1 in, 5 out]
            n201 = Read from Text File(file (use dialog)=w493, count=-1, error in=w492) -> (refnum out=w497:refnum<file>, error out=w496:errorcluster)  [unwired: 3 out]
            n202 = Close File(refnum=w497, error in=w496) -> (error out=w494:errorcluster)  [unwired: 1 out]
          }
          frame Enabled {
          }
        }
        n203 = Spreadsheet String To Array(delimiter (Tab)="", format string="", spreadsheet string="SerialPort\tCOM1\t \t \t " ("电子表格字符串"), array type (2D Dbl)=string[][] []) -> (array=w484:string[][])
        n204 = Index Array(array=w484, index (col) #1=0 ("disabled index (col)"), index (col) #2=1 ("index (col)"), index (col) #3=2 ("index (col)"), index (col) #4=3 ("index (col)"), index (col) #5=4 ("index (col)")) -> (element #1=w478:string[], element #2=w477:string[], element #3=w476:string[], element #4=w475:string[], element #5=w474:string[])  [unwired: 5 in]
      }
      event "open": Value Change {
        n205 = event-data() -> ()  [unwired: 7 out]
        n206 = call "HW File config.vi"("base path"=w514) -> ("Cancel"=w507:bool, "count"=w508:string)  [unwired: 9 out]
        n207 = case shown="假" w507 {
          tunnel: w514 -> [w537 _]
          tunnel: [w520 w543] -> w513
          tunnel: [w519 w542] -> w512
          tunnel: [w518 w541] -> w511
          tunnel: [w517 w540] -> w510
          tunnel: [w516 w539] -> w509
          tunnel: w508 -> [w515 _]
          tunnel: w506 -> [_ w543]
          tunnel: w505 -> [_ w542]
          tunnel: w504 -> [_ w541]
          tunnel: w503 -> [_ w540]
          tunnel: w502 -> [_ w539]
          frame False {
            n208 = property on="File Name" class="Str"("Value"=w515) -> ()  [unwired: 2 in, 2 out]
            n209 = Build Path(base path=w537, name or relative path=w515) -> (appended path=w536:path)
            n210 = Open/Create/Replace File(file path (use dialog)=w536) -> (refnum out=w535:refnum<file>, error out=w534:errorcluster)  [unwired: 1 in, 5 out]
            n211 = Read from Text File(file (use dialog)=w535, count=-1, error in=w534) -> (refnum out=w533:refnum<file>, text=w530:string, error out=w532:errorcluster)  [unwired: 2 out]
            n212 = Close File(refnum=w533, error in=w532) -> ()  [unwired: 2 out]
            n213 = Spreadsheet String To Array(delimiter (Tab)="", format string="", spreadsheet string=w530, array type (2D Dbl)=string[][] []) -> (array=w526:string[][])
            n214 = Index Array(array=w526, index (col) #1=0 ("disabled index (col)"), index (col) #2=1 ("index (col)"), index (col) #3=2 ("index (col)"), index (col) #4=3 ("index (col)"), index (col) #5=4 ("index (col)")) -> (element #1=w520:string[], element #2=w519:string[], element #3=w518:string[], element #4=w517:string[], element #5=w516:string[])  [unwired: 5 in]
          }
          frame True {
            n215 = property on="open" class="Bool (严格)"("Value"=FALSE) -> ()  [unwired: 2 in, 2 out]
          }
        }
        n216 = property on="Multicolumn Listbox" class="MCListbox (严格)"("Value"=0 ("Multicolumn Listbox")) -> ()  [unwired: 2 in, 2 out]
      }
    }
    "布尔" <- w82
    n217 = call "outstring.vi"("ItemNames 3"=w77, "ItemNames 2"=w76, "ItemNames 4"=w78, "ItemNames"=w71, "ItemNames 5"=w79) -> ("数组"=w70:string[], "数组 2"=w75:string[][])  [unwired: 5 in]
    n218 = Wait (ms)(milliseconds to wait=u32 20) -> ()  [unwired: 1 out]
    n219 = property on="Multicolumn Listbox" class="MCListbox (严格)"("ItemNames"=w75, "RowHdrs[]"=w70) -> ()  [unwired: 2 in, 2 out]
  }
  n220 = while {
    shift-left: _ -> [w546]
    shift-right: [w547] -> _
    shift-left: _ -> [w550]
    shift-right: ["Bar"] -> _
    tunnel: w6 -> [w551]
    stop <- w544 stop-if-true
    n221 = Not(x=w550) -> (.not. x?=w549:bool)
    n222 = Wait (ms)(milliseconds to wait=u32 10) -> ()  [unwired: 1 out]
    n223 = And(x=w549, y="Bar") -> (x .and. y?=w545:bool)
    n224 = case shown="真" "Bar" {
      tunnel: w551 -> [_ w557]
      tunnel: [w553 w556] -> w547
      tunnel: w546 -> [w553 w554]
      tunnel: w545 -> [_ w555]
      frame False {
      }
      frame True {
        n225 = case shown="假" w555 {
          tunnel: w557 -> [w563 w579]
          tunnel: [w558 w569] -> w556
          tunnel: w554 -> [w558 _]
          frame False {
            n226 = Unbundle By Name(w558) -> ("x"=w566:i16, "y"=w565:i16)
            n227 = call "Get Cursor Position.vi"() -> ("cursor position"=w568:cluster{"x":i16, "y":i16})
            n228 = Unbundle By Name(w568) -> ("x"=w567:i16, "y"=w564:i16)
            n229 = Subtract(x=w567, y=w566) -> (x-y=w560:i16)
            n230 = Subtract(x=w564, y=w565) -> (x-y=w561:i16)
            n231 = Bundle By Name(cluster=cluster{"left":i16, "top":i16} {"left"=0, "top"=0} ("new position (0,0)"), "left"=w560, "top"=w561) -> (w559:cluster{"left":i16, "top":i16})
            n232 = call "Move Window.vi"("new position (0,0)"=w559, "window refnum (NaWR)"=w563) -> ()  [unwired: 2 in, 4 out]
          }
          frame True {
            n233 = call "Get Window Rectangle.vi"("window refnum (NaWR)"=w579) -> ("window rect"=w578:T3)  [unwired: 1 in, 5 out]
            n234 = call "Extract Window Origin.vi"("window rect"=w578) -> ("window origin"=w577:cluster{"left":i16, "top":i16})  [unwired: 1 out]
            n235 = Unbundle By Name(w577) -> ("left"=w574:i16, "top"=w573:i16)
            n236 = call "Get Cursor Position.vi"() -> ("cursor position"=w576:cluster{"x":i16, "y":i16})
            n237 = Unbundle By Name(w576) -> ("x"=w575:i16, "y"=w572:i16)
            n238 = Subtract(x=w575, y=w574) -> (x-y=w570:i16)
            n239 = Subtract(x=w572, y=w573) -> (x-y=w571:i16)
            n240 = Bundle By Name(cluster=w576, "x"=w570, "y"=w571) -> (w569:cluster{"x":i16, "y":i16})
          }
        }
      }
    }
    n241 = property on="布尔" class="Bool (严格)"() -> ("Value"=w544:bool)  [unwired: 2 in, 2 out]
  }
  n242 = disable-structure shown="禁用" {
    disable-tunnel: w32 -> [w581 _]
    frame Disabled {
      n243 = control-ref of="This VI"() -> (w580:refnum<vi>)
      n244 = invoke class="VI" method="FP.Close"(reference=w580, error in=w581) -> ()  [unwired: 1 in, 3 out]
    }
    frame Enabled {
    }
  }
